vi "QueryServer_SetResponse_Query.vi"(0 "gRPCid":T1, 1 "message":string, 2 "status":i32, 3 "error in (no error)":errorcluster) -> (10 "error out":errorcluster)   [LabVIEW 2019, in "labview-grpc-query-server.lvlib"]
uses:
  labview-grpc-query-server.lvlib
  gRPC interface/Server API/typeDefs/grpcId.ctl
  QueryServer_QueryResponse.ctl
  7edc6479-9648-4038-b89b-3cf9cf8c5275.vi
  <vilib>/Utility/error.llb/Error Cluster From Error Code.vi
  gRPC interface/gprc-lvsupport.lvlib
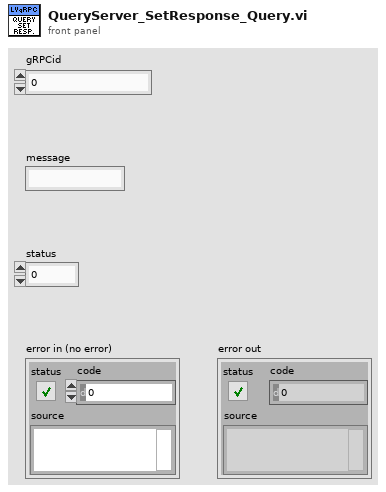
[diagram p1: front panel]
types:
  T1 = typedef "gprc-lvsupport.lvlib/grpcId.ctl" = u64
  T2 = typedef "labview-grpc-query-server.lvlib/QueryServer_QueryResponse.ctl" = cluster{"message":string, "status":i32}
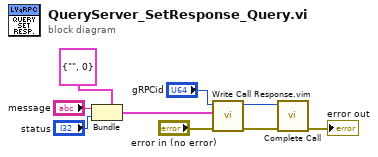
[diagram p0: block diagram]
diagram:
  n1 = Bundle(cluster=T2 {"message"="", "status"=0} ("QueryResponse"), "message"="message", "status"="status") -> (w3:T2)
  n2 = call "Write Call Response.vim"("error in (no error)"="error in (no error)", "Response Data"=w3, "gRPCid in"="gRPCid") -> ("error out"=w5:errorcluster, "gRPCid"=w4:T1)  [unwired: 7 in]
  n3 = call "Complete Call.vi"("gRPCid"=w4, "error in (no error)"=w5) -> ("error out"=→"error out":errorcluster)  [unwired: 8 in]
